vi "Control_iTC.vi"() -> ()   [LabVIEW 2015]
panel:
  out "String 2":string
  out "Communication":string
  in  "Record new values":bool
  out "Heater Voltage (V)":dbl
  out "Temperature (K)":dbl
  out "Set Point (T)":dbl
  out "Automatic Mode":i8(ring) items=["OFF", "ON"]
  in  "error in (no error)":errorcluster
  out "error out":errorcluster
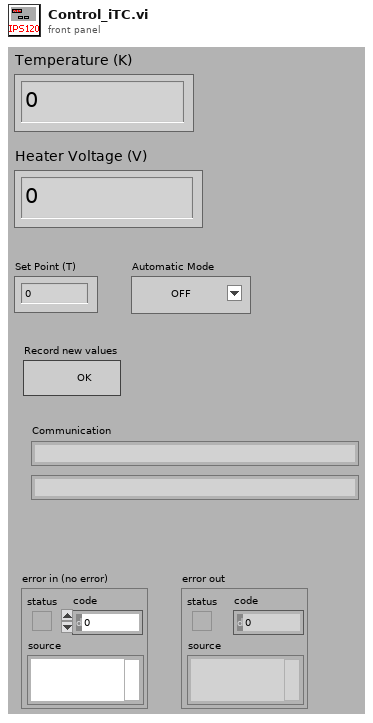
[diagram p1: front panel]
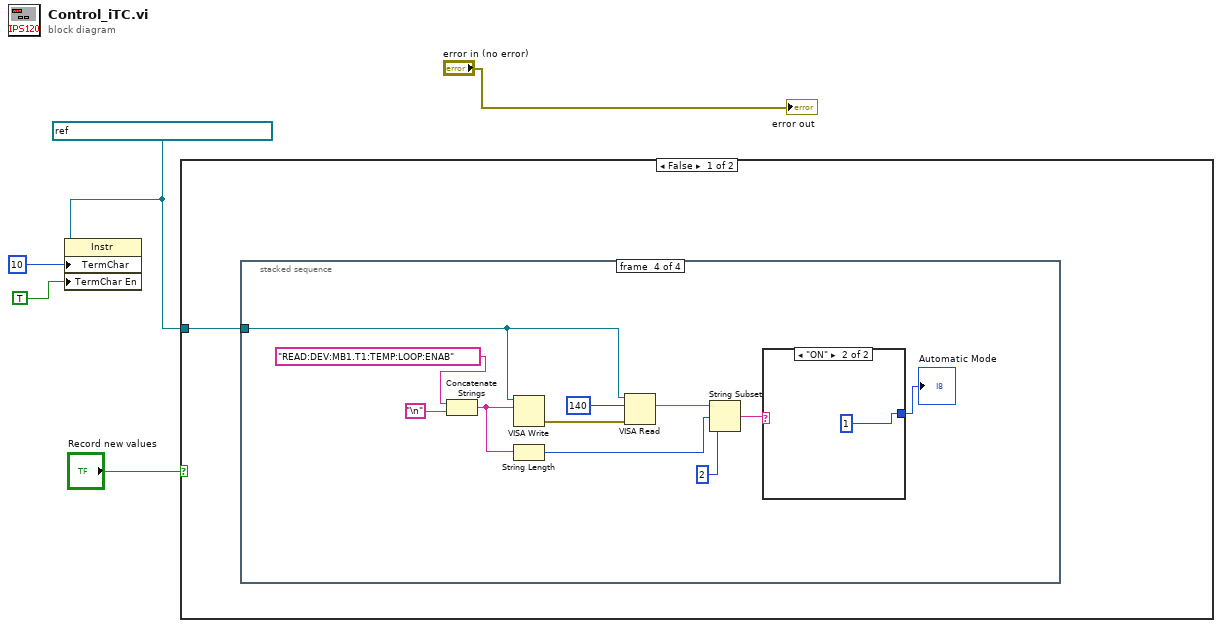
[diagram p0: block diagram]
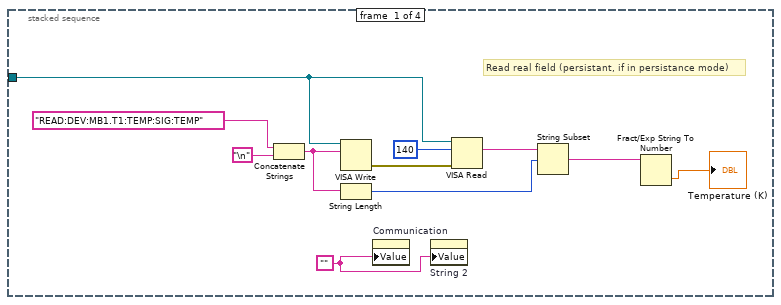
[diagram p2: hidden frame]
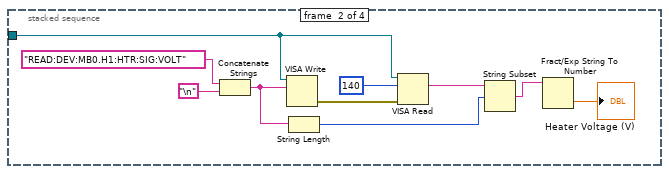
[diagram p3: hidden frame]
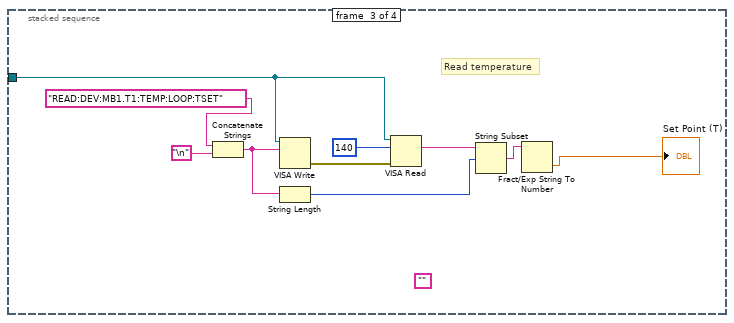
[diagram p4: hidden frame]
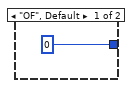
[diagram p5: hidden frame]
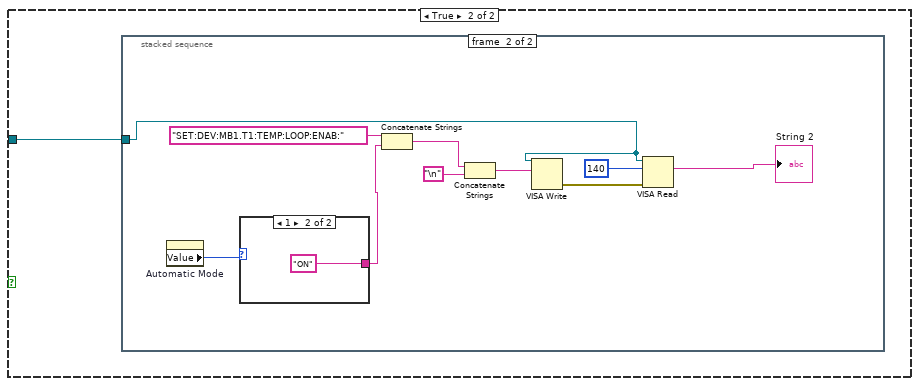
[diagram p6: hidden frame]
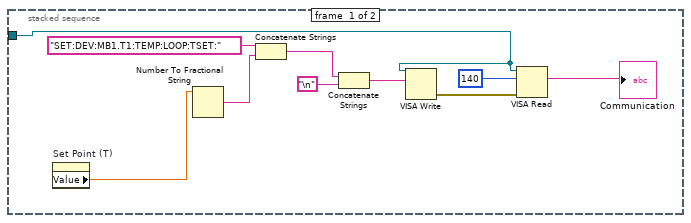
[diagram p7: hidden frame]
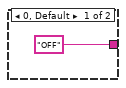
[diagram p8: hidden frame]
diagram:
  w2 = refnum<visa-resource-name> "TCPIP0::192.168.128.2::7020::SOCKET" ("VISA resource name")
  n1 = property class="Instr"(reference=w2, "TermChar"=10, "TermChar En"=TRUE) -> ()  [unwired: 1 in, 2 out]
  n2 = case shown="False" "Record new values" {
    tunnel: w2 -> [w6 w51]
    frame False {
      n3 = stacked-sequence {
        tunnel: w6 -> [w8 w18 w28 w41]
        frame #0 {
          w7 = ""
          # "Read real field (persistant, if in persistance mode)"
          n4 = Concatenate Strings("READ:DEV:MB1.T1:TEMP:SIG:TEMP" ("string"), "\n") -> (w10:string)
          n5 = VISA Write(VISA resource name=w8, write buffer=w10) -> (error out=w16:errorcluster)  [unwired: 1 in, 2 out]
          n6 = String Length(string=w10) -> (length=w11:i32)
          n7 = property on="Communication" class="Str"("Value"=w7) -> ()  [unwired: 2 in, 2 out]
          n8 = property on="String 2" class="Str"("Value"=w7) -> ()  [unwired: 2 in, 2 out]
          n9 = VISA Read(VISA resource name=w8, byte count=140, error in (no error)=w16) -> (read buffer=w12:string)  [unwired: 3 out]
          n10 = String Subset(string=w12, offset (0)=w11) -> (substring=w9:string)  [unwired: 1 in]
          n11 = Fract/Exp String To Number(string=w9) -> (number=→"Temperature (K)":dbl)  [unwired: 3 in, 1 out]
        }
        frame #1 {
          n12 = Concatenate Strings("READ:DEV:MB0.H1:HTR:SIG:VOLT" ("string"), "\n") -> (w22:string)
          n13 = VISA Write(VISA resource name=w18, write buffer=w22) -> (error out=w26:errorcluster)  [unwired: 1 in, 2 out]
          n14 = String Length(string=w22) -> (length=w20:i32)
          n15 = VISA Read(VISA resource name=w18, byte count=140, error in (no error)=w26) -> (read buffer=w21:string)  [unwired: 3 out]
          n16 = String Subset(string=w21, offset (0)=w20) -> (substring=w19:string)  [unwired: 1 in]
          n17 = Fract/Exp String To Number(string=w19) -> (number=→"Heater Voltage (V)":dbl)  [unwired: 3 in, 1 out]
        }
        frame #2 {
          (unwired) ""
          # "Read temperature"
          n18 = Concatenate Strings("READ:DEV:MB1.T1:TEMP:LOOP:TSET" ("string"), "\n") -> (w30:string)
          n19 = VISA Write(VISA resource name=w28, write buffer=w30) -> (error out=w36:errorcluster)  [unwired: 1 in, 2 out]
          n20 = String Length(string=w30) -> (length=w31:i32)
          n21 = VISA Read(VISA resource name=w28, byte count=140, error in (no error)=w36) -> (read buffer=w32:string)  [unwired: 3 out]
          n22 = String Subset(string=w32, offset (0)=w31) -> (substring=w29:string)  [unwired: 1 in]
          n23 = Fract/Exp String To Number(string=w29) -> (number=→"Set Point (T)":dbl)  [unwired: 3 in, 1 out]
        }
        frame #3 {
          n24 = Concatenate Strings("READ:DEV:MB1.T1:TEMP:LOOP:ENAB" ("string"), "\n") -> (w42:string)
          n25 = VISA Write(VISA resource name=w41, write buffer=w42) -> (error out=w48:errorcluster)  [unwired: 1 in, 2 out]
          n26 = String Length(string=w42) -> (length=w43:i32)
          n27 = VISA Read(VISA resource name=w41, byte count=140, error in (no error)=w48) -> (read buffer=w44:string)  [unwired: 3 out]
          n28 = String Subset(string=w44, offset (0)=w43, length (rest)=2) -> (substring=w40:string)
          n29 = case shown="\"ON\"" w40 {
            tunnel: [0 1] -> w39
            frame "OF", Default {
            }
            frame "ON" {
            }
          }
          "Automatic Mode" <- w39
        }
      }
    }
    frame True {
      n30 = stacked-sequence {
        tunnel: w51 -> [w54 w63]
        frame #0 {
          n31 = property on="Set Point (T)" class="DigNum (strict)"() -> ("Value"=w53:dbl)  [unwired: 2 in, 2 out]
          n32 = Number To Fractional String(number=w53) -> (F-format string=w60:string)  [unwired: 3 in]
          n33 = Concatenate Strings("SET:DEV:MB1.T1:TEMP:LOOP:TSET:" ("string"), w60) -> (w55:string)
          n34 = Concatenate Strings(w55, "\n") -> (w56:string)
          n35 = VISA Write(VISA resource name=w54, write buffer=w56) -> (error out=w59:errorcluster)  [unwired: 1 in, 2 out]
          n36 = VISA Read(VISA resource name=w54, byte count=140, error in (no error)=w59) -> (read buffer=→"Communication":string)  [unwired: 3 out]
        }
        frame #1 {
          n37 = property on="Automatic Mode" class="Ring (strict)"() -> ("Value"=w65:i8)  [unwired: 2 in, 2 out]
          n38 = case shown="1" w65 {
            tunnel: ["OFF" "ON"] -> w64
            frame 0, Default {
            }
            frame 1 {
            }
          }
          n39 = Concatenate Strings("SET:DEV:MB1.T1:TEMP:LOOP:ENAB:" ("string"), w64) -> (w66:string)
          n40 = Concatenate Strings(w66, "\n") -> (w67:string)
          n41 = VISA Write(VISA resource name=w63, write buffer=w67) -> (error out=w70:errorcluster)  [unwired: 1 in, 2 out]
          n42 = VISA Read(VISA resource name=w63, byte count=140, error in (no error)=w70) -> (read buffer=→"String 2":string)  [unwired: 3 out]
        }
      }
    }
  }
  "error out" <- "error in (no error)"
